vi "ASM.Boom.vi"(8 "error in (no error)":errorcluster, 11 "AsmTestMachine in":refnum<class "AsmTestMachine.lvclass">) -> (0 "error out":errorcluster, 3 "AsmTestMachine out":refnum<class "AsmTestMachine.lvclass">)   [LabVIEW 2021, in "AsmTestMachine.lvlib" / "AsmTestMachine.lvclass"]
uses:
  AsmTestMachine.lvclass
  AsmTestMachine.lvclass/AsmTestMachine.ctl
  Source/ActorStateMachine/ActorStateMachine/ActorStateMachine.lvclass
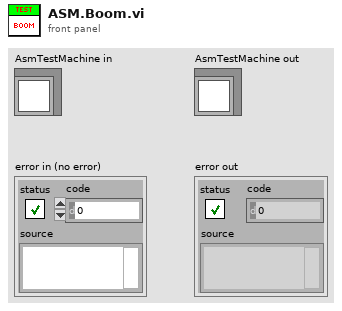
[diagram p1: front panel]
types:
  T1 = enum32{"Invalid", "Standard", "Closed", "Hidden", "Minimized", "Maximized"}
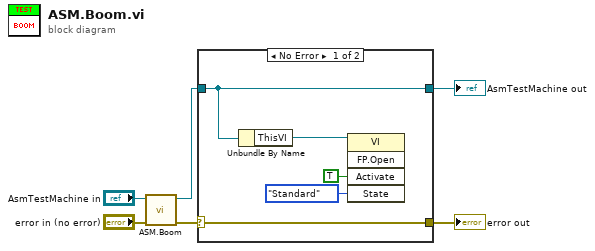
[diagram p0: block diagram]
diagram:
  n1 = call-parent "ASM.Boom.vi"("error in (no error)"="error in (no error)", "ActorStateMachine in"="AsmTestMachine in") -> ("error out"=w4:errorcluster, "ActorStateMachine out"=w2:refnum<class "AsmTestMachine.lvclass">)  [unwired: 8 in]
  n2 = case shown="No Error" w4 {
    selector: w4 -> [w11 w13]
    tunnel: [w11 w13] -> w3
    tunnel: [w10 w12] -> w1
    tunnel: w2 -> [w10 w12]
    frame No Error {
      n3 = Unbundle By Name(w10) -> ("ThisVI"=w9:refnum<vi>)
      n4 = invoke class="VI" method="FP.Open"(reference=w9, "Activate"=TRUE ("Activate?"), "State"=T1."Standard") -> ()  [unwired: 2 in, 5 out]
    }
    frame Error {
    }
  }
  "error out" <- w3
  "AsmTestMachine out" <- w1
